vi "Load TabAcqType index.vi"(8 "error in (no error)":errorcluster, 11 "S4GUI in":refnum<class "S4GUI.lvclass">) -> (0 "error out":errorcluster, 3 "S4GUI out":refnum<class "S4GUI.lvclass">)   [LabVIEW 2018, in "S4GUI.lvclass"]
uses:
  S4GUI.lvclass
  S4GUI.lvclass/S4GUI.ctl
  <vilib>/Utility/config.llb/Read Key (U32).vi
  <vilib>/Utility/config.llb/NI_LVConfig.lvlib
panel:
  out "file created?":bool
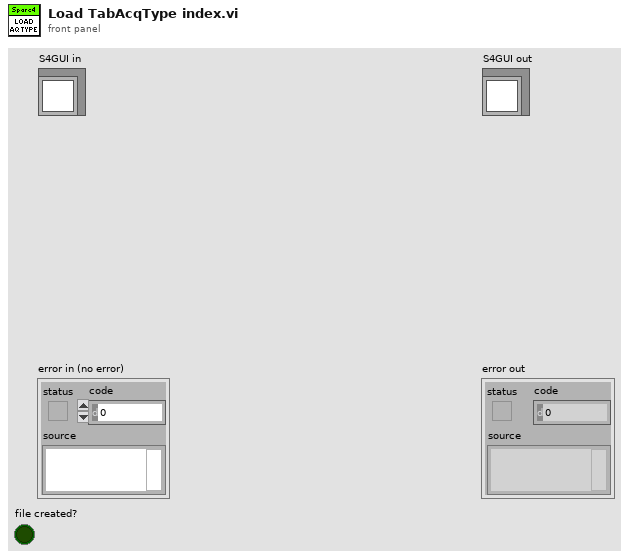
[diagram p1: front panel]
types:
  T1 = typedef "NI_LVConfig.lvlib/Config Data RefNum.ctl" = refnum<k1>
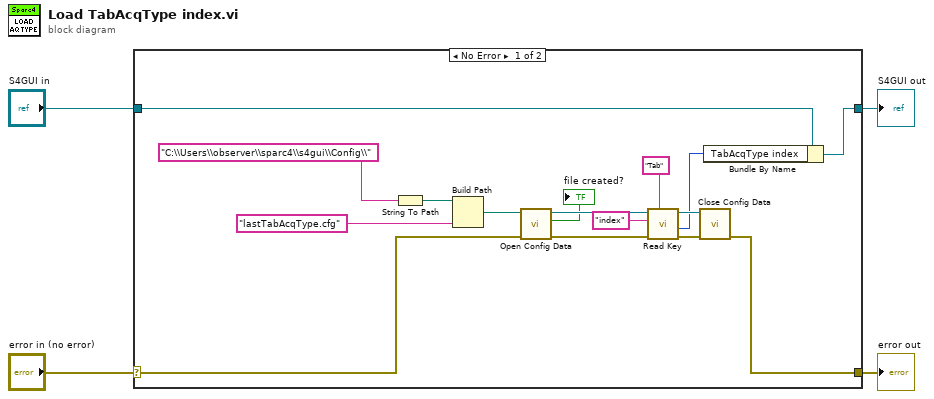
[diagram p0: block diagram]
diagram:
  n1 = case shown="No Error" "error in (no error)" {
    selector: "error in (no error)" -> [w10 w22]
    tunnel: [w9 w22] -> w3
    tunnel: [w6 w21] -> w1
    tunnel: "S4GUI in" -> [w7 w21]
    frame No Error {
      n2 = String To Path(string="C:\\Users\\observer\\sparc4\\s4gui\\Config\\") -> (path=w13:path)
      n3 = Build Path(base path=w13, name or relative path="lastTabAcqType.cfg") -> (appended path=w20:path)
      n4 = call <vilib>:"Open Config Data.vi"("error in (no error)"=w10, "configuration file path"=w20) -> ("error out"=w17:errorcluster, "file created?"=→"file created?":bool, "refnum"=w19:T1)  [unwired: 7 in]
      n5 = call-poly <vilib>:"Read Key.vi"("section"="Tab", "error in (no error)"=w17, "key"="index", "refnum"=w19) -> ("error out"=w14:errorcluster, "value"=w5:u32, "refnum out"=w15:T1)  [unwired: 4 in, 1 out]
      n6 = call <vilib>:"Close Config Data.vi"("error in (no error)"=w14, "refnum"=w15) -> ("error out"=w9:errorcluster)  [unwired: 8 in, 1 out]
      n7 = Bundle By Name(cluster=w7, "TabAcqType index"=w5) -> (w6:refnum<class "S4GUI.lvclass">)
    }
    frame Error {
    }
  }
  "error out" <- w3
  "S4GUI out" <- w1
